vi "LWXPS_ZygoSetOffsetX.vi"(6 "LabVIEW error IN":errorcluster, 8 "Offset value for X":i64, 9 "XPS Reference IN":refnum<k24>) -> (0 "LabVIEW error OUT":errorcluster, 1 "XPS Error String":string, 2 "Returned error code":i32, 3 "XPS Reference OUT":refnum<k24>)   [LabVIEW 2014]
uses:
  D:/XPSQ8_LabView_Library/Development/Source/Dll/Newport.XPS.CommandInterface.dll
  Dll/Newport.XPS.CommandInterface.dll
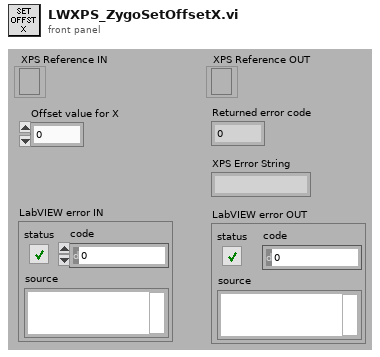
[diagram p1: front panel]
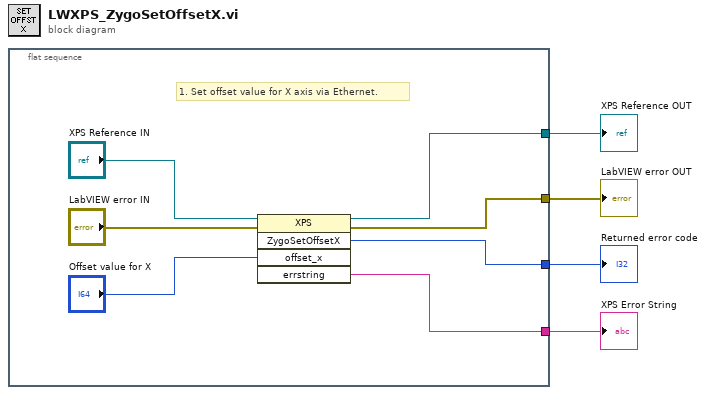
[diagram p0: block diagram]
diagram:
  n1 = flat-sequence {
    tunnel: [w9] -> w4
    tunnel: [w7] -> w3
    tunnel: [w10] -> w2
    tunnel: [w6] -> w1
    frame #0 {
      # "1. Set offset value for X axis via Ethernet."
      n2 = invoke class="XPS" method="ZygoSetOffsetX"(reference="XPS Reference IN", error in="LabVIEW error IN", "offset_x"="Offset value for X") -> (reference out=w9:refnum<k24>, error out=w7:errorcluster, "ZygoSetOffsetX"=w10:i32, "errstring"=w6:string)  [unwired: 2 in, 1 out]
    }
  }
  "XPS Reference OUT" <- w4
  "LabVIEW error OUT" <- w3
  "Returned error code" <- w2
  "XPS Error String" <- w1
